vi "Reverse Plot Order.vi"(8 "error in (no error)":errorcluster, 11 "Graph Manager in":refnum<class "Graph Manager.lvclass">) -> (0 "error out":errorcluster, 3 "Graph Manager out":refnum<class "Graph Manager.lvclass">)   [LabVIEW 2013, in "Graph Manager.lvclass"]
uses:
  Graph Manager.lvclass
  Graph Manager.lvclass/Graph Manager.ctl
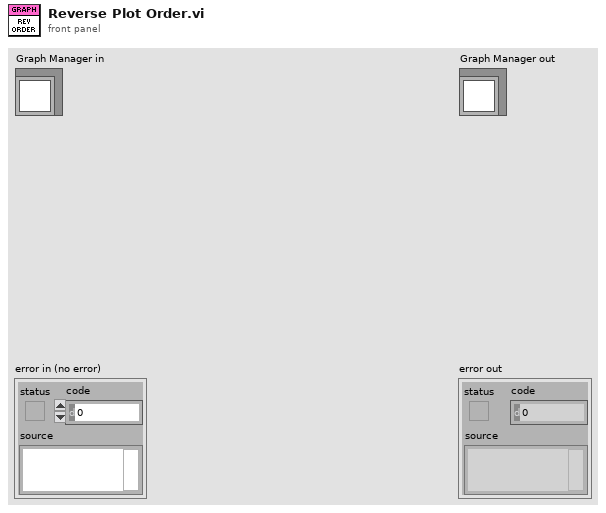
[diagram p1: front panel]
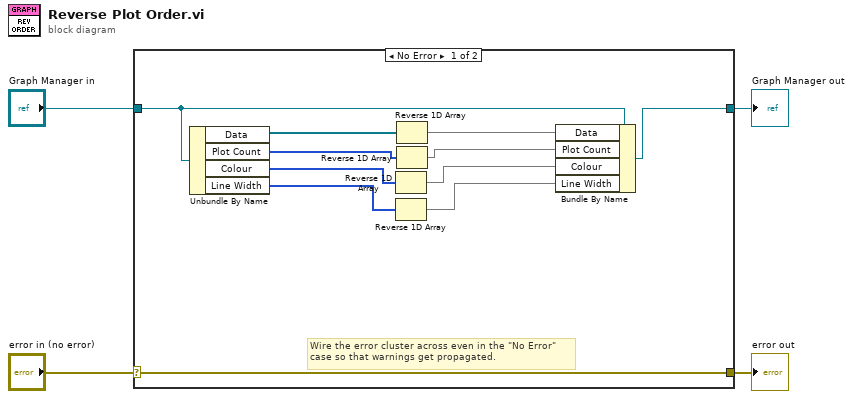
[diagram p0: block diagram]
diagram:
  n1 = case shown="No Error" "error in (no error)" {
    selector: "error in (no error)" -> [w15 w17]
    tunnel: [w15 w17] -> w3
    tunnel: [w13 w16] -> w1
    tunnel: "Graph Manager in" -> [w14 w16]
    frame No Error {
      # "Wire the error cluster across even in the \"No Error\"\ncase so that warnings get propagated."
      n2 = Unbundle By Name(w14) -> ("Data"=w12:refnum<data-value>[], "Plot Count"=w10:i32[], "Colour"=w9:u32[], "Line Width"=w8:u8[])
      n3 = Reverse 1D Array(array=w9) -> (reversed array=w6:u32[])
      n4 = Reverse 1D Array(array=w8) -> (reversed array=w7:u8[])
      n5 = Reverse 1D Array(array=w12) -> (reversed array=w11:refnum<data-value>[])
      n6 = Reverse 1D Array(array=w10) -> (reversed array=w5:i32[])
      n7 = Bundle By Name(cluster=w14, "Data"=w11, "Plot Count"=w5, "Colour"=w6, "Line Width"=w7) -> (w13:refnum<class "Graph Manager.lvclass">)
    }
    frame Error {
    }
  }
  "error out" <- w3
  "Graph Manager out" <- w1
